vi "workinglogic.vi"() -> ()   [LabVIEW 2025]
panel:
  out "data out":string
  out "value":dbl
  out "command":string
  in  "stop":bool
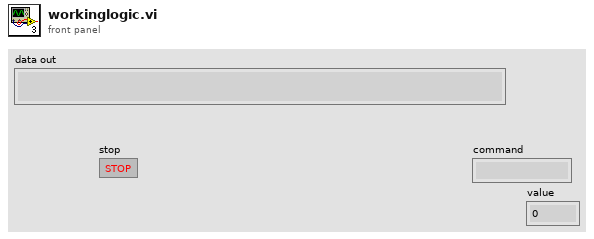
[diagram p1: front panel]
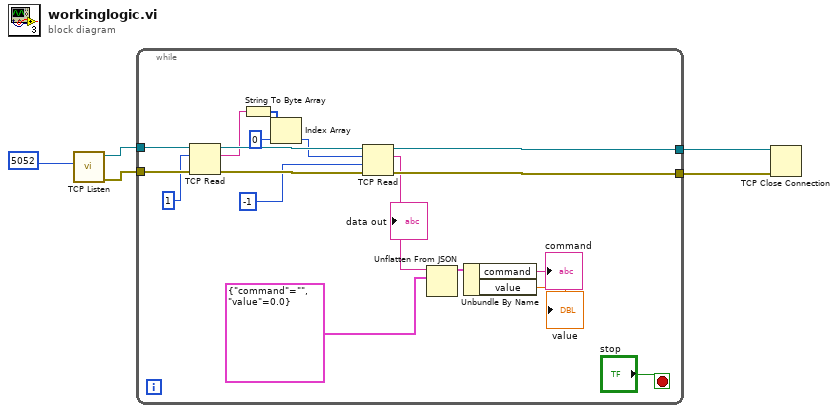
[diagram p0: block diagram]
diagram:
  n1 = call <vilib>:"TCP Listen.vi"("port"=u16 5052) -> ("error out"=w4:errorcluster, "connection ID"=w5:refnum<k5>)  [unwired: 6 in, 3 out]
  n2 = while {
    tunnel: w5 -> [w23]
    tunnel: w4 -> [w21]
    tunnel: [w17] -> w2
    tunnel: [w16] -> w1
    stop <- "stop" stop-if-true
    n3 = TCP Read(connection ID=w23, bytes to read=1, error in (no error)=w21) -> (connection ID out=w22:refnum<k5>, data out=w9:string, error out=w20:errorcluster)  [unwired: 2 in]
    n4 = String To Byte Array(string=w9) -> (unsigned byte array=w8:u8[])
    n5 = Index Array(array=w8, index=0) -> (element=w6:u8)
    n6 = TCP Read(connection ID=w22, bytes to read=w6, error in (no error)=w20, 9:-1 ("timeout ms (25000)")) -> (connection ID out=w16:refnum<k5>, data out=w14:string, error out=w17:errorcluster)  [unwired: 1 in]
    "data out" <- w14
    n7 = Unflatten From JSON(JSON string=w14, type and defaults=cluster{"command":string, "value":dbl} {"command"="", "value"=0.0}) -> (value=w12:cluster{"command":string, "value":dbl})  [unwired: 5 in, 1 out]
    n8 = Unbundle By Name(w12) -> ("command"=→"command":string, "value"=→"value":dbl)
  }
  n9 = TCP Close Connection(connection ID=w1, error in (no error)=w2) -> ()  [unwired: 1 in, 2 out]
